vi "CheezyMxatan.vi"(1 "arg":dbl) -> (0 "mxatan(arg)":dbl)   [LabVIEW 2015]
uses:
  <userlib>/836-Library/CheezyMath/MathConstantsNames.ctl
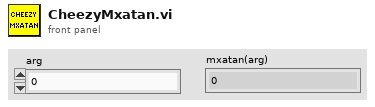
[diagram p1: front panel]
types:
  T1 = typedef "MathConstantsNames.ctl" = enum16{"sq2p1", "sq2m1", "p4", "p3", "p2", "p1", "p0", "q4", "q3", "q2", "q1", "q0", "PIO2"}
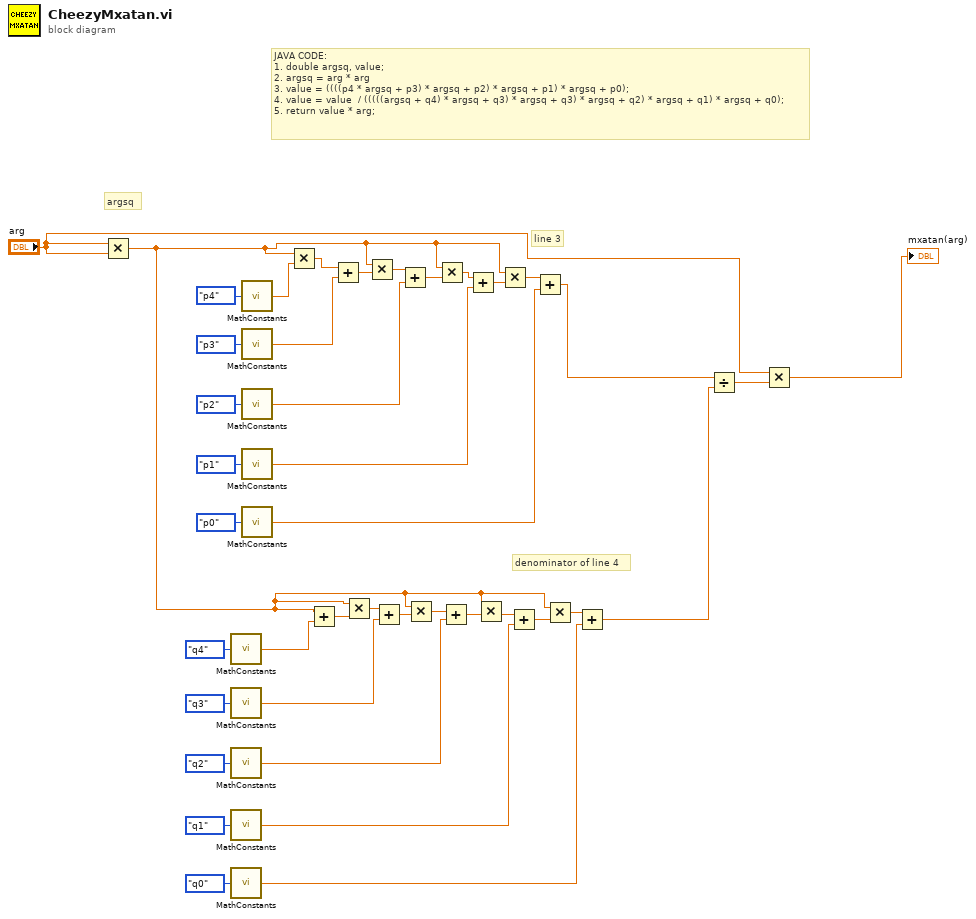
[diagram p0: block diagram]
diagram:
  # "denominator of line 4"
  # "line 3"
  # "JAVA CODE:\n1. double argsq, value;\n2. argsq = arg * arg\n3. value = ((((p4 * argsq + p3) * argsq + p2) * argsq + p1) * argsq + p0);\n4. value = value  / (((((argsq + q4) * argsq + q3) * argsq + q3) * argsq + q2) * argsq + q1) * argsq + q0);\n5. return value * arg;"
  # "argsq"
  n1 = Multiply(x="arg", y="arg") -> (x*y=w8:dbl)
  n2 = call <userlib>:"MathConstants.vi"("Constant Name"=MathConstantsNames."q4") -> ("Constant Value"=w19:dbl)
  n3 = call <userlib>:"MathConstants.vi"("Constant Name"=MathConstantsNames."q3") -> ("Constant Value"=w16:dbl)
  n4 = call <userlib>:"MathConstants.vi"("Constant Name"=MathConstantsNames."q2") -> ("Constant Value"=w13:dbl)
  n5 = call <userlib>:"MathConstants.vi"("Constant Name"=MathConstantsNames."q1") -> ("Constant Value"=w10:dbl)
  n6 = call <userlib>:"MathConstants.vi"("Constant Name"=MathConstantsNames."q0") -> ("Constant Value"=w6:dbl)
  n7 = call <userlib>:"MathConstants.vi"("Constant Name"=MathConstantsNames."p4") -> ("Constant Value"=w31:dbl)
  n8 = call <userlib>:"MathConstants.vi"("Constant Name"=MathConstantsNames."p3") -> ("Constant Value"=w29:dbl)
  n9 = call <userlib>:"MathConstants.vi"("Constant Name"=MathConstantsNames."p2") -> ("Constant Value"=w26:dbl)
  n10 = call <userlib>:"MathConstants.vi"("Constant Name"=MathConstantsNames."p1") -> ("Constant Value"=w23:dbl)
  n11 = call <userlib>:"MathConstants.vi"("Constant Name"=MathConstantsNames."p0") -> ("Constant Value"=w20:dbl)
  n12 = Multiply(x=w8, y=w31) -> (x*y=w30:dbl)
  n13 = Add(x=w8, y=w19) -> (x+y=w18:dbl)
  n14 = Add(x=w30, y=w29) -> (x+y=w28:dbl)
  n15 = Multiply(x=w8, y=w18) -> (x*y=w17:dbl)
  n16 = Multiply(x=w8, y=w28) -> (x*y=w27:dbl)
  n17 = Add(x=w17, y=w16) -> (x+y=w15:dbl)
  n18 = Add(x=w27, y=w26) -> (x+y=w25:dbl)
  n19 = Multiply(x=w8, y=w15) -> (x*y=w14:dbl)
  n20 = Multiply(x=w8, y=w25) -> (x*y=w24:dbl)
  n21 = Add(x=w14, y=w13) -> (x+y=w12:dbl)
  n22 = Add(x=w24, y=w23) -> (x+y=w22:dbl)
  n23 = Multiply(x=w8, y=w12) -> (x*y=w11:dbl)
  n24 = Multiply(x=w8, y=w22) -> (x*y=w21:dbl)
  n25 = Add(x=w11, y=w10) -> (x+y=w9:dbl)
  n26 = Add(x=w21, y=w20) -> (x+y=w5:dbl)
  n27 = Multiply(x=w8, y=w9) -> (x*y=w7:dbl)
  n28 = Add(x=w7, y=w6) -> (x+y=w4:dbl)
  n29 = Divide(x=w5, y=w4) -> (x/y=w3:dbl)
  n30 = Multiply(x="arg", y=w3) -> (x*y=→"mxatan(arg)":dbl)
